vi "Example Switch Socket.vi"() -> ()   [LabVIEW 2013]
uses:
  C:/tf/play/labview/Tinkerforge.dll
panel:
  in  "uid":string="amb"
  in  "port":i32=4223
  in  "host":string="localhost"
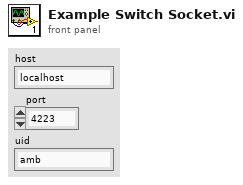
[diagram p1: front panel]
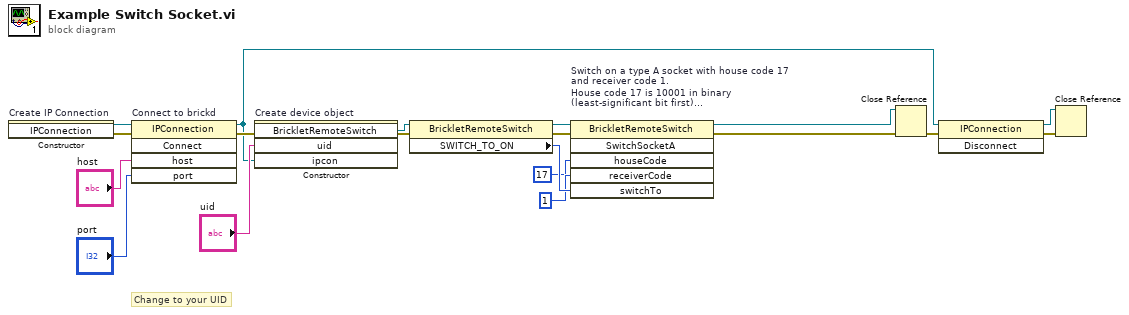
[diagram p0: block diagram]
diagram:
  # "Change to your UID"
  n1 = constructor on="Create IP Connection" class="IPConnection"() -> (reference out=w19:refnum<k24>, error out=w8:errorcluster)  [unwired: 3 in, 1 out]
  n2 = invoke on="Connect to brickd" class="IPConnection" method="Connect"(reference=w19, error in=w8, "host"="host", "port"="port") -> (reference out=w10:refnum<k24>, error out=w15:errorcluster)  [unwired: 1 in, 3 out]
  n3 = constructor on="Create device object" class="BrickletRemoteSwitch"(error in=w15, "uid"="uid", "ipcon"=w10) -> (error out=w7:errorcluster, "BrickletRemoteSwitch"=w4:refnum<k24>)  [unwired: 2 in, 3 out]
  n4 = property class="BrickletRemoteSwitch"(reference=w4, error in=w7) -> (reference out=w5:refnum<k24>, error out=w6:errorcluster, "SWITCH_TO_ON"=w3:u8)
  n5 = invoke on="Switch on a type A socket with house code 17 and receiver code 1.\nHouse code 17 is 10001 in binary (least-significant bit first)\nand means that the DIP switches 1 and 5 are on and 2-4 are off.\nReceiver code 1 is 10000 in binary (least-significant bit first)\nand means that the DIP switch A is on and B-E are off." class="BrickletRemoteSwitch" method="SwitchSocketA"(reference=w5, error in=w6, "houseCode"=u8 17, "receiverCode"=u8 1, "switchTo"=w3) -> (reference out=w13:refnum<k24>, error out=w14:errorcluster)  [unwired: 1 in, 4 out]
  n6 = Close Reference(reference=w13, error in (no error)=w14) -> (error out=w12:errorcluster)
  n7 = invoke class="IPConnection" method="Disconnect"(reference=w10, error in=w12) -> (reference out=w9:refnum<k24>, error out=w11:errorcluster)  [unwired: 1 in, 1 out]
  n8 = Close Reference(reference=w9, error in (no error)=w11) -> ()  [unwired: 1 out]
